vi "My timer.vi"(0 "Target Time Sec":dbl, 1 "Reset":bool, 2 "Pause":bool, 3 "error in (no error)":errorcluster) -> (7 "Remaining Time":dbl, 8 "Elapsed Time":dbl, 9 "Time Expired":bool, 10 "error out":errorcluster)   [LabVIEW 2012]
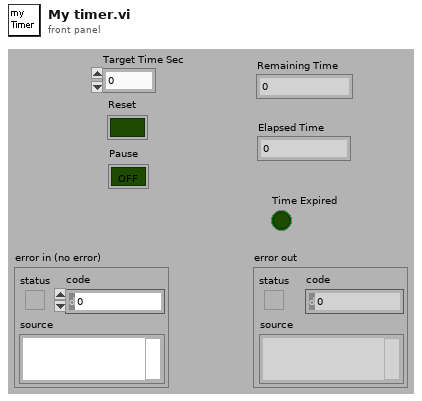
[diagram p1: front panel]
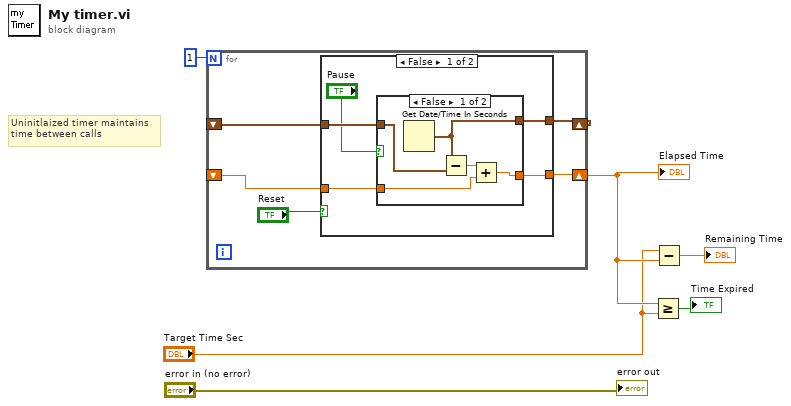
[diagram p0: block diagram]
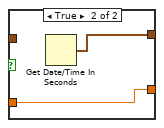
[diagram p2: hidden frame]
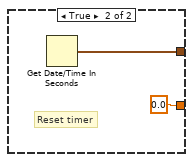
[diagram p3: hidden frame]
diagram:
  # "Uninitlaized timer maintains\ntime between calls"
  n1 = for {
    N: 1 -> [_]
    shift-right: [w11] -> _
    shift-left: _ -> [w10]
    shift-right: [w8] -> w2
    shift-left: _ -> [w9]
    n2 = case shown="False" "Reset" {
      tunnel: [w16 w25] -> w11
      tunnel: w10 -> [w15 _]
      tunnel: w9 -> [w14 _]
      tunnel: [w12 0.0] -> w8
      frame False {
        n3 = case shown="False" "Pause" {
          tunnel: [w20 w23] -> w16
          tunnel: w15 -> [w21 _]
          tunnel: [w17 w22] -> w12
          tunnel: w14 -> [w18 w22]
          frame False {
            n4 = Get Date/Time In Seconds() -> (seconds since 1Jan1904=w20:timestamp)
            n5 = Subtract(x=w20, y=w21) -> (x-y=w19:dbl)
            n6 = Add(x=w19, y=w18) -> (x+y=w17:dbl)
          }
          frame True {
            n7 = Get Date/Time In Seconds() -> (seconds since 1Jan1904=w23:timestamp)
          }
        }
      }
      frame True {
        # "Reset timer"
        n8 = Get Date/Time In Seconds() -> (seconds since 1Jan1904=w25:timestamp)
      }
    }
  }
  "Elapsed Time" <- w2
  n9 = Greater Or Equal?(x=w2, y="Target Time Sec") -> (x >= y?=→"Time Expired":bool)
  n10 = Subtract(x="Target Time Sec", y=w2) -> (x-y=→"Remaining Time":dbl)
  "error out" <- "error in (no error)"
